vi "Handle Nested Error.vi"(8 "error in (no error)":errorcluster, 9 "Error to Handle":errorcluster, 11 "Actor ErrorStop in":refnum<class "Actor ErrorStop.lvclass">) -> (0 "error out":errorcluster, 3 "Actor ErrorStop out":refnum<class "Actor ErrorStop.lvclass">)   [LabVIEW 2012, in "Actor ErrorStop.lvlib" / "Actor ErrorStop.lvclass"]
uses:
  Actor ErrorStop.lvclass
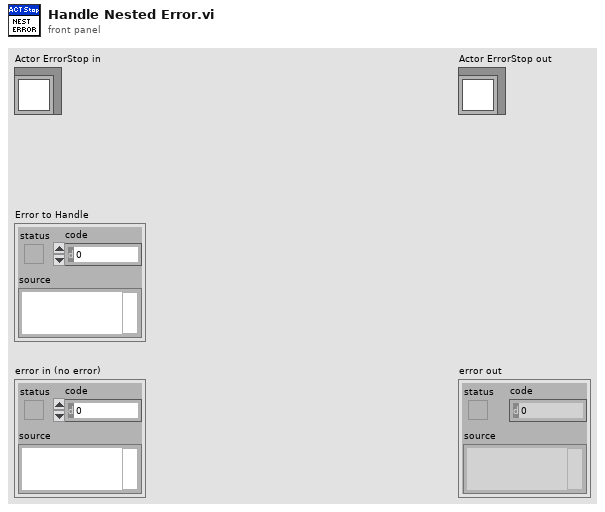
[diagram p1: front panel]
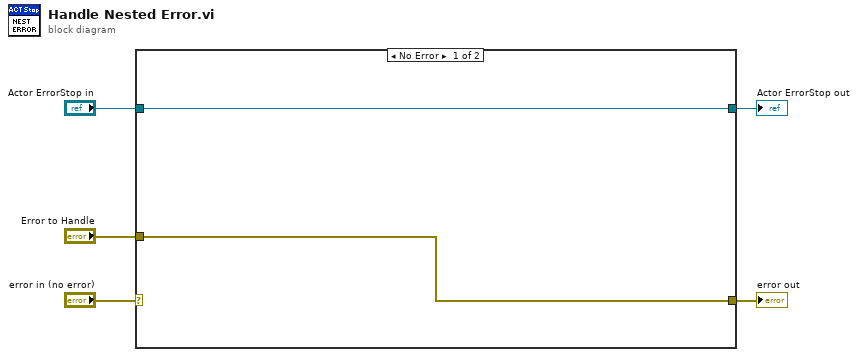
[diagram p0: block diagram]
diagram:
  n1 = case shown="No Error" "error in (no error)" {
    selector: "error in (no error)" -> [_ w9]
    tunnel: [w6 w9] -> w5
    tunnel: [w7 w8] -> w3
    tunnel: "Actor ErrorStop in" -> [w7 w8]
    tunnel: "Error to Handle" -> [w6 _]
    frame No Error {
    }
    frame Error {
    }
  }
  "error out" <- w5
  "Actor ErrorStop out" <- w3
